vi "Autotuning Smith Predictor.vi"() -> ()   [LabVIEW 2023]
doc: "This example demonstrates how to use a PID Autotuning for systems with large delay, by using the Internal Model Control algorithm for first order model with delay."
uses:
  <vilib>/addons/control/pid/NI_PID_autopid.lvlib
panel:
  in  "Instructions":string="Overview: This example demonstrates how to use a PID Autotuning for systems with large delay, by using the Internal Model Control algorithm for first-order model with transport delay (deadtime).\nInstructions:\n1. Run the VI and wait until the process variable (PV) reaches near setpoint (SP).\n2.  On the PID Autotuning Design section, select the  type of controller, step amplitude for the 'open loop step response'. Then, press Identify and tune to start the process.\n3.  When the tuned PID gains do not change anymore or the indicator tuning completed? flashes, the identification is done and you can accept new gains by pressing Accept gain. That will transfer the new gain to PID Gains.\n4. Click Identify and tune again to go back to the automatic control. You can try different options and repeat this process. Time constant factor specifies a divider to apply to the identified time constant to obtain the desired time constant response. Time constant factor to a value greater than 1 makes the desired time constant used in the design faster (more aggressive). Time constant factor to a value less than 1 makes the response slower (more conservative).\nStep amplitude specifies the amplitude of the step applied to the open loop identification.  \n5. Click Stop to stop the VI.\n"
  out "tuned PID gains":T1={"proportional gain (Kc)"=15.221889907608013, "integral time (Ti, min)"=0.002027201803862475, "derivative time (Td, min)"=0.0002815558060920104} {"derivative time (Td, min)" format="%#.6g"; "integral time (Ti, min)" format="%#.6g"; "proportional gain (Kc)" format="%#.6g"}
  in  "Accept gain":bool
  in  "Alpha":dbl(slide) scale=0.0..1.0
  out "tuning completed?":bool
  in  "initial plant parameters":T2={"process gain"=2.515490777679412, "time constant (s)"=2.529236380296785, "delay time (s)"=2.5407395402910935} {"delay time (s)" format="%.3f"; "time constant (s)" format="%.3f"; "process gain" format="%.3f"}
  in  "Automatic":bool=TRUE
  in  "Reinitialize":bool
  in  "autotuning parameters":T3={"type of controller"=1, "time constant factor"=2.0, "step amplitude"=1.0} {"time constant factor" scale=0.0001..1000.0; "step amplitude" format="%.2f"; "type of controller" items=["P", "PI", "PID"]}
  out "MV":dbl(graph)=20.39115328927357
  in  "Identify and tune":bool
  in  "SP1:":dbl(slide)=37.254901960784316 min=0.0 max=0.0 scale=0.0..100.0
  in  "MV1:":dbl(slide)=15.081495361740814 scale=-100.0..100.0
  out "PV1:":dbl(slide)=42.840793682454986 scale=0.0..100.0
  in  "PID Gains":T1={"proportional gain (Kc)"=1.0198114826651394, "integral time (Ti, min)"=0.06332676917403887, "derivative time (Td, min)"=0.0} {"derivative time (Td, min)" format="%#.6g"; "integral time (Ti, min)" format="%#.6g"; "proportional gain (Kc)" format="%#.6g"}
  in  "Sampling Time dt (s)":dbl=0.1 min=0.001 step=0.01 format="%#.3p"
  in  "Stop":bool
  out "SP and PV":cluster{"initial PV":dbl, "SP1:":dbl}(graph)={"initial PV"=50.98160323470328, "SP1:"=50.98039215686275}
  # "Proportional-Integral-Derivative (PID) Controller"
  # "PID Autotuning Design"
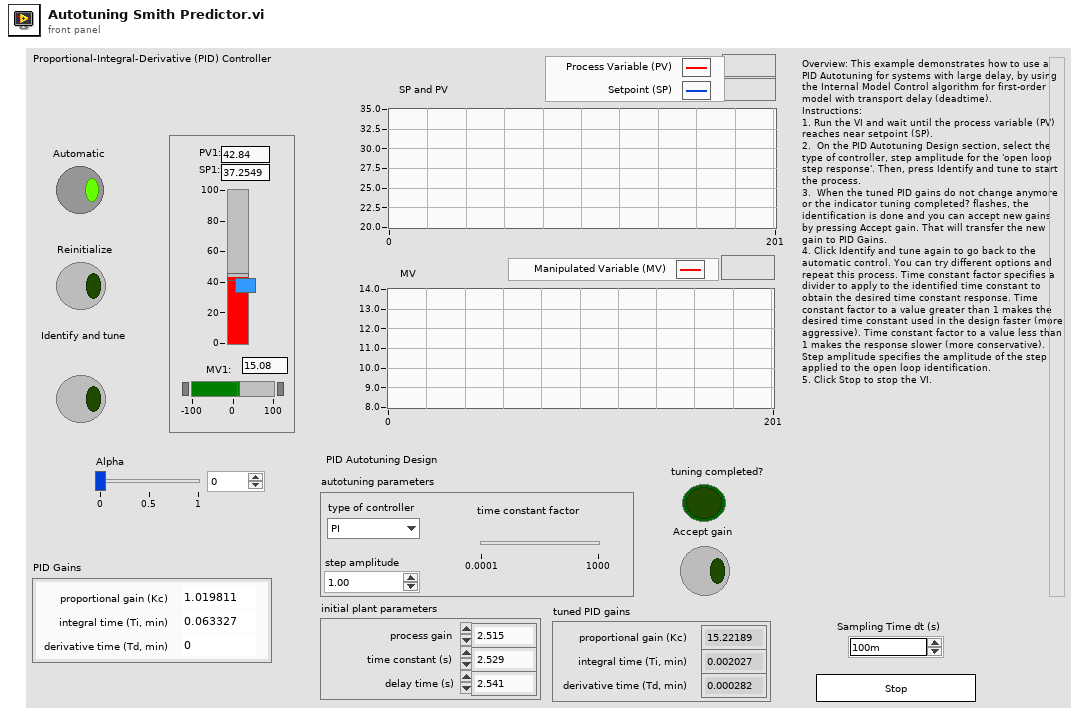
[diagram p1: front panel]
types:
  T1 = cluster{"proportional gain (Kc)":dbl, "integral time (Ti, min)":dbl, "derivative time (Td, min)":dbl}
  T2 = cluster{"process gain":dbl, "time constant (s)":dbl, "delay time (s)":dbl}
  T3 = cluster{"type of controller":u16, "time constant factor":dbl, "step amplitude":dbl}
  T4 = cluster{"static gain":dbl, "lag (s)":dbl, "deadtime (s)":dbl, "load":dbl, "deadband":dbl, "sensor noise":dbl, "initial PV":dbl, "plant noise":dbl}
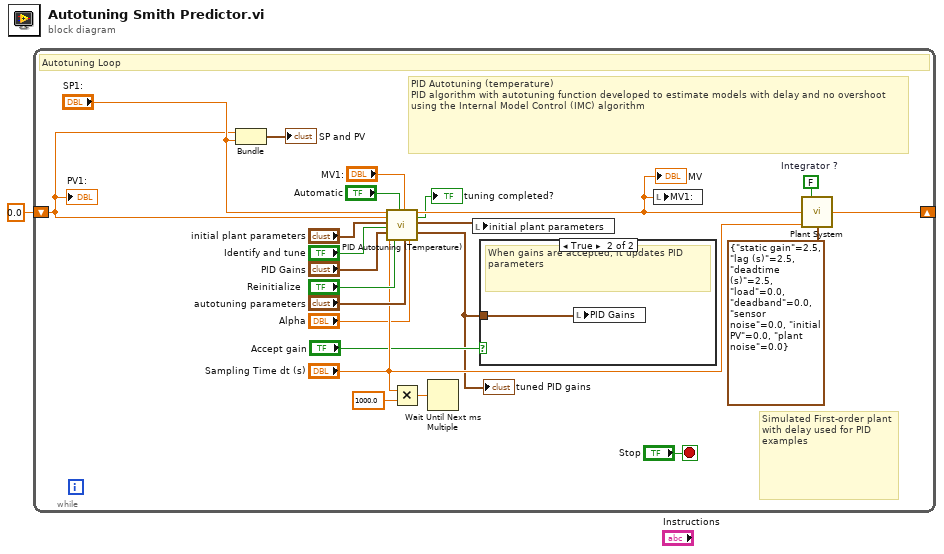
[diagram p0: block diagram]
diagram:
  n1 = while {
    shift-right: [w2] -> _
    shift-left: 0.0 ("Plant Output") -> [w3]
    stop <- "Stop" stop-if-true
    w13 = FALSE  # Integrator ?
    # "PID Autotuning (temperature)\nPID algorithm with autotuning function developed to estimate models with delay and no overshoot using the Internal Model Control (IMC) algorithm"
    # "Simulated First-order plant with delay used for PID examples"
    # "Autotuning Loop"
    n2 = Bundle("Plant Output"=w3, "SP1:"="SP1:") -> (→"SP and PV":cluster{"Plant Output":dbl, "SP1:":dbl})  [unwired: 1 in]
    n3 = call <vilib>:"PID Autotuning (Temperature).vi"("desired temperature"="SP1:", "measured temperature"=w3, "plant parameters in"="initial plant parameters", "autotune? (F)"="Identify and tune", "PID gains in"="PID Gains", "dt (s)"="Sampling Time dt (s)", "reinitialize? (F)"="Reinitialize", "auto? (T)"="Automatic", "manual control"="MV1:", "autotuning parameters"="autotuning parameters", "alpha"="Alpha") -> ("output"=w17:dbl, "tuning completed?"=→"tuning completed?":bool, "plant parameters out"=w11:T2, "PID gains out"=w6:T1)  [unwired: 5 in]
    "MV" <- w17
    "tuned PID gains" <- w6
    n4 = Multiply(x="Sampling Time dt (s)", y=1000.0 ("Numeric")) -> (x*y=w5:dbl)
    n5 = Wait Until Next ms Multiple(millisecond multiple=w5) -> ()  [unwired: 1 out]
    n6 = local write "initial plant parameters"(w11) -> ()
    n7 = case shown="True" "Accept gain" {
      tunnel: w6 -> [_ w25]
      frame False {
        # "otherwise, do nothing"
      }
      frame True {
        # "When gains are accepted, it updates PID parameters"
        n8 = local write "PID Gains"(w25) -> ()
      }
    }
    n9 = local write "MV1:"(w17) -> ()
    n10 = call "Plant System.vi"("Integrator ?"=w13, "Plant Input"=w17, "dt (s)"="Sampling Time dt (s)", "process parameters"=T4 {"static gain"=2.5, "lag (s)"=2.5, "deadtime (s)"=2.5, "load"=0.0, "deadband"=0.0, "sensor noise"=0.0, "initial PV"=0.0, "plant noise"=0.0} ("plant parameters")) -> ("Plant Output"=w2:dbl)  [unwired: 11 in]
    "PV1:" <- w3
  }
